vi "Actuator and Pump Control Phases Main Prog.vi"() -> ()   [LabVIEW 2020]
uses:
  Controls/Pump Phases.ctl
  Controls/SImulation Data.ctl
  <vilib>/Instr/_visa.llb/VISA Open Access Mode.ctl
  <vilib>/Instr/_visa.llb/VISA Configure Serial Port (Instr).vi
  <vilib>/Utility/file.llb/Read Delimited Spreadsheet (string).vi
  <vilib>/Utility/file.llb/Write Delimited Spreadsheet (string).vi
  SubVIs/Pump Global Variables.vi
panel:
  in  "Clear Simulation Data":bool
  in  "stop 3":bool
  out "error out 5":errorcluster
  out "VISA resource name out 3":refnum<visa-resource-name>
  out "error out 4":errorcluster
  out "VISA resource name out 2":refnum<visa-resource-name>
  out "Valve error out":errorcluster
  out "Valve resource name out":refnum<visa-resource-name>
  out "read buffer":string
  in  "Volume Dis Update":bool
  out "Dispensed":string
  out "Extracted Numbers":dbl[](array[numeric]) format="%#.6g"
  in  "Simulation data":T1[](array[typedef]) {"Time Stamp" format="%<%.3X>T"}
  out "Elapsed Time (s)":dbl
  out "Time":timestamp=timestamp(3688120494.225 s since 1904-01-01)
  in  "stop 2":bool
  in  "State?":bool
  in  "Pump Phases Path":path
  out "source 2":string
  out "code 2":i32
  out "status 2":bool
  out "source":string
  out "code":i32
  out "status":bool
  in  "Save Simulation Data":bool
  in  "Save Pump Phases":bool
  in  "Load Pump Phases":bool
  in  "Save Basic Param":bool
  out "Complete":bool[](array[boolean])
  out "Busy":bool caption="BUSY"
  in  "Add":bool
  in  "Update":bool
  in  "Delete last":bool
  in  "Delete unselected":bool
  in  "Select":bool[](array[boolean])=[TRUE, TRUE, TRUE, TRUE, TRUE, TRUE, TRUE, TRUE, TRUE, TRUE, TRUE, TRUE, TRUE]
  out "Direction1":string caption="Direction"
  out "Rate1":string caption="Rate"
  out "Target1":string caption="Target"
  in  "RUN":bool
  in  "Serial Reset":bool
  in  "Reset1":bool
  in  "Send":bool
  in  "Units":string(combo)="mm"
  in  "Pump Direction":string(combo)="wdr"
  in  "Incr/Decr Time (S)":dbl
  in  "Diameter (mm)":dbl=20.5 min=0.1 max=50.0
  in  "Array of Pump Phases":T2[](array[typedef]) {"Valve Position" min=0 max=10 step=1; "Pump Rate" format="%#_4g"}
  out "Max rate":dbl format="%#_4g"
  out "Min rate":dbl format="%#_4g"
  in  "Pump Serial Port":refnum<visa-resource-name>="COM1"
  in  "stop":bool
  out "error out 2":cluster{}
  in  "Valve VISA resource name":refnum<visa-resource-name>="COM2"
  out "error out":cluster{}
  in  "Send/read":bool
  in  "Stop":bool=TRUE
  out "Read Buffer":string
  in  "Valve Command":string="/?"
  in  "Valve Control":T3(radio)=enum."SetR1"
  out "Numeric":i32
  out "Bytes at Port":u32
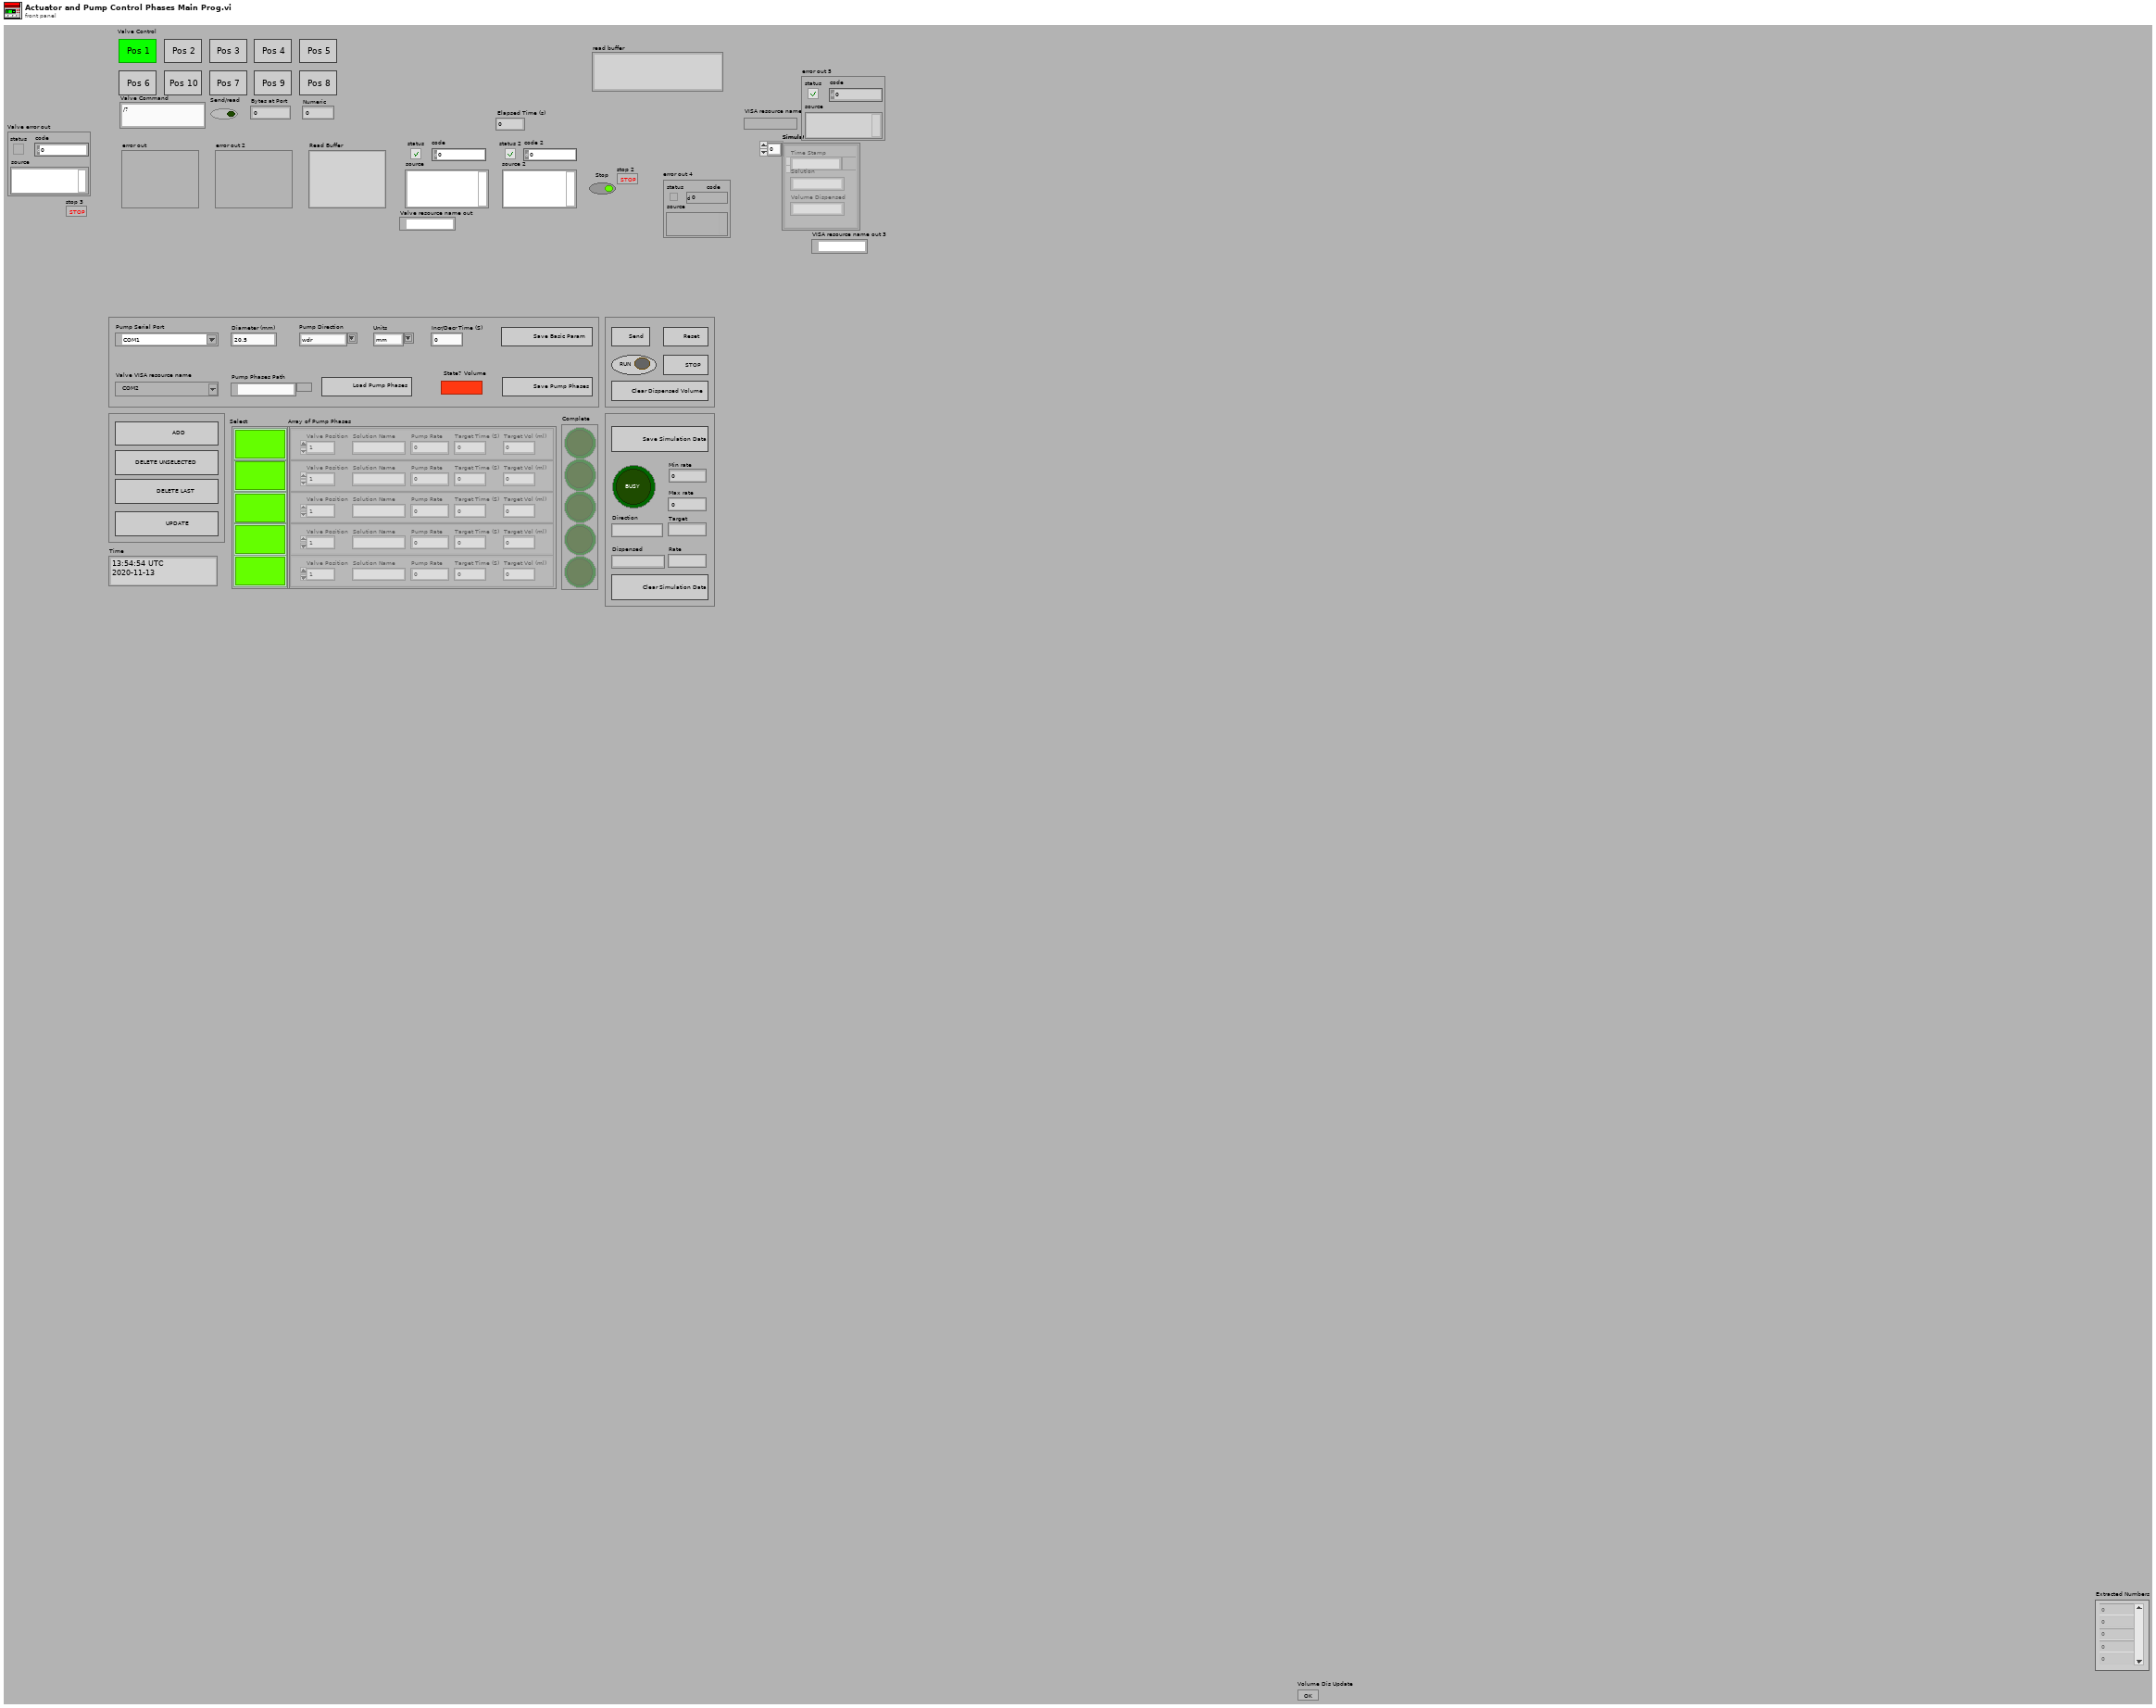
[diagram p1: front panel]
types:
  T1 = typedef "SImulation Data.ctl" = cluster{"Time Stamp":timestamp, "Solution":string, "Volume Dispensed":string}
  T2 = typedef "Pump Phases.ctl" = cluster{"Valve Position":sgl, "Solution Name":string, "Pump Rate":dbl, "Target Time":dbl, "Target Volume":dbl}
  T3 = enum32{"No Selection", "SetR1", "SetR2", "SetR3", "SetR4", "SetR6", "SetR7", "SetR8", "SetR9", "SetR10", "SetR5"}
  T4 = enum8{"Enabled", "Disabled", "Disabled and Grayed Out"}
  T5 = typedef "VISA Open Access Mode.ctl" = u32
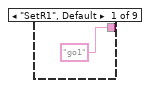
[diagram p2: hidden frame]
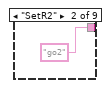
[diagram p3: hidden frame]
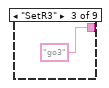
[diagram p4: hidden frame]
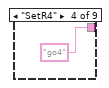
[diagram p5: hidden frame]
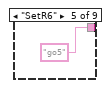
[diagram p6: hidden frame]
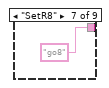
[diagram p7: hidden frame]
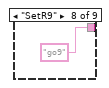
[diagram p8: hidden frame]
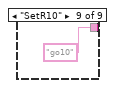
[diagram p9: hidden frame]
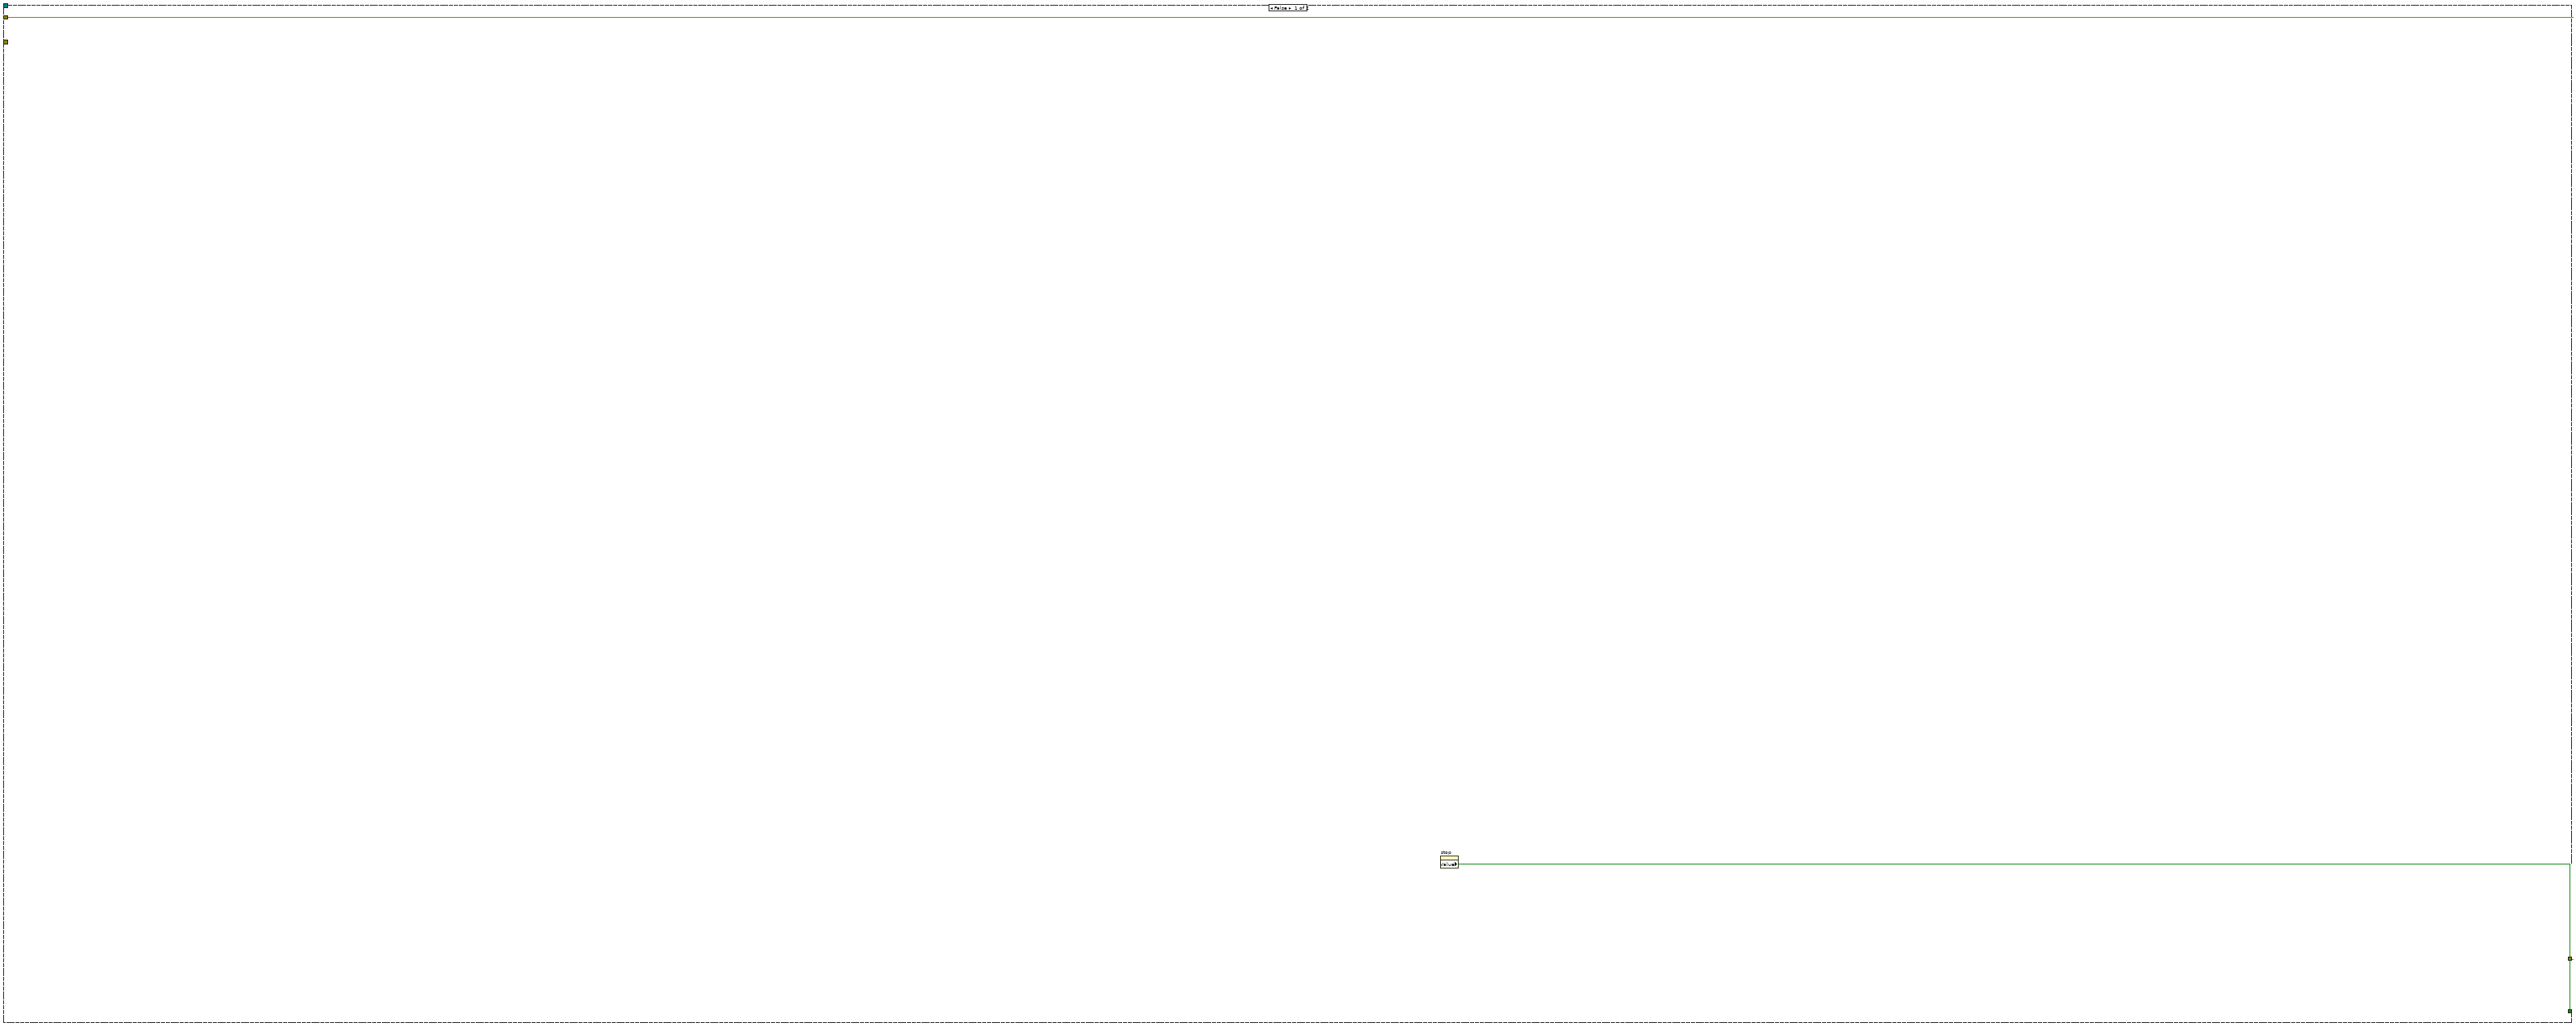
[diagram p13: hidden frame]
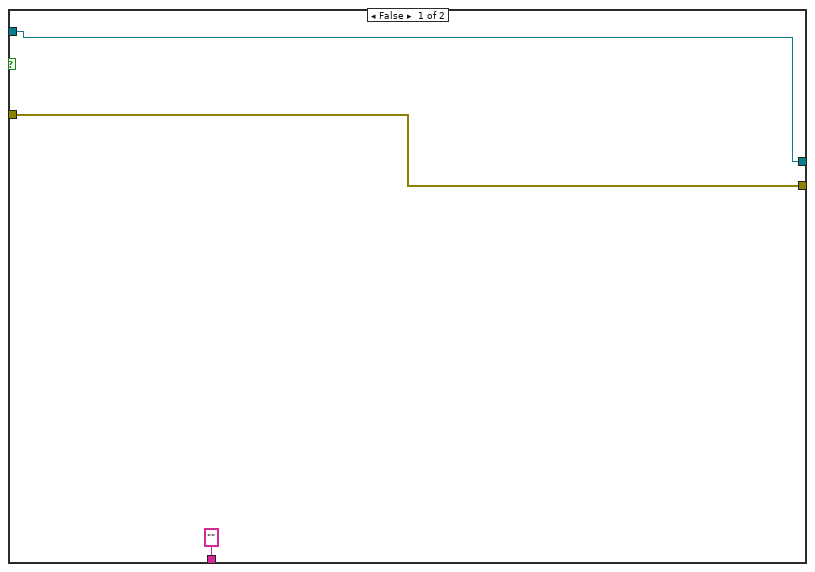
[diagram p14: hidden frame]
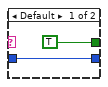
[diagram p15: hidden frame]
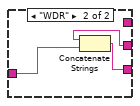
[diagram p16: hidden frame]
diagram:
  n1 = local read "Array of Pump Phases"() -> (w5:T2[])
  n2 = while {
    stop <- "stop 2" stop-if-true
    n3 = call "Elapsed Time"() -> ("Elapsed Time (s)"=→"Elapsed Time (s)":dbl)  [unwired: 12 in, 7 out]
    n4 = Get Date/Time In Seconds() -> (seconds since 1Jan1904=w10:timestamp)
    "Time" <- w10
    n5 = Get Date/Time String(seconds (now)=w10) -> ()  [unwired: 2 in, 2 out]
  }
  n6 = Array Size(array=w5) -> (size(s)=w3:i32)
  n7 = Equal To 0?(x=w3) -> (x = 0?=w4:bool)
  n8 = case shown="True" w4 {
    frame False {
    }
    frame True {
      n9 = Initialize Array(T2 {"Valve Position"=1.0, "Solution Name"="", "Pump Rate"=0.0, "Target Time"=0.0, "Target Volume"=0.0} ("Cluster"), 1 ("dimension size")) -> (w12:T2[])
      n10 = local write "Array of Pump Phases"(w12) -> ()
    }
  }
  n11 = Initialize Array(FALSE, w3) -> (w6:bool[])
  n12 = local write "Complete"(w6) -> ()
  n13 = while {
    tunnel: [w16] -> w8
    tunnel: [w19] -> w2
    tunnel: [w18] -> w1
    stop <- w16 stop-if-true
    w21 = T5 0 items=["VISA Defaults"=0, "Exclusive Lock"=1, "Load Configured Settings"=4] ("Access Mode")
    n14 = VISA Open(access mode=w21, VISA resource name="Valve VISA resource name") -> (VISA resource name=w22:refnum<visa-resource-name>, error out=w24:errorcluster)  [unwired: 3 in]
    n15 = Decimal String To Number(string="9600" ("Baud Rate"), default (0L)=u32 0 ("default (0 I32)")) -> (number=w29:u32)  [unwired: 1 in, 1 out]
    n16 = call-poly "VISA Configure Serial Port"("VISA resource name"="Pump Serial Port", "termination char\n(0xA = '\\n' = LF)"=u8 13 ("termination char\n(0xA = '\\n' = LF)"), "Enable Termination\nChar (T)"=TRUE ("Enable Termination\nChar (T)"), "baud rate (9600)"=w29) -> ("VISA resource name out"=w17:refnum<visa-resource-name>, "error out"=w15:errorcluster)  [unwired: 10 in]
    n17 = call-poly "VISA Configure Serial Port"("VISA resource name"=w22, "Enable Termination\nChar (T)"=FALSE ("Enable Termination\nChar (T)"), "error in (no error)"=w24) -> ("VISA resource name out"=w19:refnum<visa-resource-name>, "error out"=w18:errorcluster)  [unwired: 11 in]
    n18 = Unbundle By Name(w15) -> ("status"=w26:bool)
    n19 = Not(x=w26) -> (.not. x?=w25:bool)
    n20 = case shown="True" w25 {
      tunnel: w17 -> [_ w37]
      tunnel: w15 -> [w35 w42]
      tunnel: [w34 w41] -> w16
      tunnel: [w35 w40] -> w27
      tunnel: w19 -> [_ w39]
      tunnel: w18 -> [_ w38]
      tunnel: w15 -> [_ w36]
      frame False {
        n21 = property on="stop" class="Bool (strict)"() -> ("Value"=w34:bool)  [unwired: 2 in, 2 out]
      }
      frame True {
        n22 = while {
          tunnel: w42 -> [w109]
          tunnel: w37 -> [w110]
          tunnel: [w121] -> w46
          tunnel: [w120] -> w45
          tunnel: ["stop"] -> w41
          tunnel: w39 -> [w111]
          tunnel: w38 -> [w101]
          stop <- w136 stop-if-true
          n23 = Wait Until Next ms Multiple(millisecond multiple=u32 50) -> ()  [unwired: 1 out]
          n24 = global read "Pump Global Variables.vi" "Diameter (mm)"() -> (w126:dbl)
          n25 = case shown="True" "Send" {
            tunnel: w110 -> [w387 w398]
            tunnel: w109 -> [w386 w397]
            tunnel: [w387 w395] -> w108
            tunnel: [w386 w396] -> w107
            tunnel: "Pump Direction" -> [_ w394]
            frame False {
            }
            frame True {
              n26 = flat-sequence {
                tunnel: w398 -> [w403]
                tunnel: w397 -> [w402]
                tunnel: [w400] -> w393
                tunnel: [w399] -> w391
                tunnel: w393 -> [w411]
                tunnel: [w411] -> w392
                tunnel: w391 -> [w410]
                tunnel: [w410] -> w390
                tunnel: w392 -> [w414]
                tunnel: w390 -> [w413]
                tunnel: w394 -> [w412]
                tunnel: [w416] -> w389
                tunnel: [w415] -> w388
                tunnel: [w421] -> w395
                tunnel: [w422] -> w396
                tunnel: w389 -> [w422]
                tunnel: w388 -> [w421]
                frame #0 {
                  n27 = local read "Diameter (mm)"() -> (w405:dbl)
                  n28 = Number To Fractional String(number=w405, precision (6)=i16 2) -> (F-format string=w404:string)  [unwired: 2 in]
                  n29 = Concatenate Strings("dia" ("string"), w404, "\r") -> (w401:string)
                  n30 = VISA Write(VISA resource name=w403, write buffer=w401, error in (no error)=w402) -> (VISA resource name out=w400:refnum<visa-resource-name>, error out=w399:errorcluster)  [unwired: 1 out]
                }
                frame #1 {
                  n31 = Wait (ms)(milliseconds to wait=u32 100) -> ()  [unwired: 1 out]
                }
                frame #2 {
                  n32 = Concatenate Strings("dir" ("string"), w412, "\r") -> (w419:string)
                  n33 = VISA Write(VISA resource name=w414, write buffer=w419, error in (no error)=w413) -> (VISA resource name out=w415:refnum<visa-resource-name>, error out=w416:errorcluster)  [unwired: 1 out]
                }
                frame #3 {
                  n34 = Wait (ms)(milliseconds to wait=u32 100) -> ()  [unwired: 1 out]
                }
              }
            }
          }
          n35 = case shown="True" "Add" {
            frame False {
            }
            frame True {
              n36 = flat-sequence {
                frame #0 {
                  n37 = local read "Array of Pump Phases"() -> (w472:T2[])
                  n38 = Build Array (concatenate)(w472, T2 {"Valve Position"=1.0, "Solution Name"="", "Pump Rate"=0.0, "Target Time"=0.0, "Target Volume"=0.0} ("Cluster")) -> (w470:T2[])
                  n39 = local write "Array of Pump Phases"(w470) -> ()
                }
                frame #1 {
                  n40 = local write "Update"(TRUE) -> ()
                }
              }
            }
          }
          n41 = case shown="True" "Delete last" {
            frame False {
            }
            frame True {
              n42 = flat-sequence {
                frame #0 {
                  n43 = local read "Array of Pump Phases"() -> (w499:T2[])
                  n44 = Delete From Array(array=w499, length=1) -> (array with subset deleted=w500:T2[])  [unwired: 1 in, 1 out]
                  n45 = local write "Array of Pump Phases"(w500) -> ()
                }
                frame #1 {
                  n46 = local write "Update"(TRUE) -> ()
                }
              }
            }
          }
          n47 = case shown="False" "State?" {
            frame False {
              n48 = property on="Target Volume" class="DigNum (strict)"("DisabledEnum"=T4."Enabled" ("Disabled")) -> ()  [unwired: 2 in, 2 out]
              n49 = property on="Target Time" class="DigNum (strict)"("DisabledEnum"=T4."Disabled and Grayed Out" ("Disabled")) -> ()  [unwired: 2 in, 2 out]
            }
            frame True {
              n50 = property on="Target Volume" class="DigNum (strict)"("DisabledEnum"=T4."Disabled and Grayed Out" ("Disabled")) -> ()  [unwired: 2 in, 2 out]
              n51 = property on="Target Time" class="DigNum (strict)"("DisabledEnum"=T4."Enabled" ("Disabled")) -> ()  [unwired: 2 in, 2 out]
            }
          }
          n52 = feedback-in #1("RUN") -> ()
          n53 = feedback #1() -> (w129:bool)  [unwired: 1 in]
          n54 = formula code="r=p*((d/20)**2)*5.1;"("d"=w126, "p"=3.141592653589793) -> ("r"=w134:dbl)
          n55 = global read "Pump Global Variables.vi" "Units 2"() -> (w113:string)
          n56 = case shown="True" "Update" {
            frame False {
            }
            frame True {
              n57 = local read "Array of Pump Phases"() -> (w493:T2[])
              n58 = local write "Update"(FALSE ("Update")) -> ()
              n59 = Array Size(array=w493) -> (size(s)=w492:i32)
              n60 = Greater Than 0?(x=w492) -> (x > 0?=w491:bool)
              n61 = case shown="True" w491 {
                frame False {
                }
                frame True {
                  n62 = local read "Array of Pump Phases"() -> (w498:T2[])
                  n63 = Array Size(array=w498) -> (size(s)=w495:i32)
                  n64 = property on="Select" class="Arr (strict)"("Number of Rows"=w495) -> ()  [unwired: 2 in, 2 out]
                  n65 = property on="Array of Pump Phases" class="Arr (strict)"("Number of Rows"=w495) -> ()  [unwired: 2 in, 2 out]
                  n66 = property on="Complete" class="Arr (strict)"("Number of Rows"=w495) -> ()  [unwired: 2 in, 2 out]
                  n67 = Initialize Array(FALSE, w495) -> (w496:bool[])
                  n68 = local write "Complete"(w496) -> ()
                }
              }
            }
          }
          n69 = case shown="\"mh\"" w113 {
            tunnel: w134 -> [w576 w578 w582 w586 w587]
            tunnel: [w575 w579 w581 w586 w587] -> w131
            frame "mh" {
              n70 = Multiply(x=w576, y=60.0) -> (x*y=w575:dbl)
            }
            frame "um" {
              n71 = Multiply(x=1000.0, y=w578) -> (x*y=w579:dbl)
            }
            frame "uh" {
              n72 = Multiply(x=1000.0, y=60.0) -> (x*y=w585:dbl)
              n73 = Multiply(x=w585, y=w582) -> (x*y=w581:dbl)
            }
            frame Default {
            }
            frame "mm" {
            }
          }
          "Max rate" <- w131
          n74 = disable-structure shown="Disabled" {
            disable-tunnel: w129 -> [w339 _]
            disable-tunnel: "RUN" -> [w336 _]
            frame Disabled {
              n75 = Build Array(w336, w339) -> (w340:bool[])
              n76 = Boolean Array To Number(Boolean array=w340) -> (number=w341:u32)
              n77 = call <vilib>:"Trim Whitespace.vi"("string"="0") -> ("trimmed string"=w338:string)  [unwired: 1 in]
              n78 = case shown="1" w341 {
                tunnel: [w343 w347 w372] -> _
                tunnel: [w342 w346 w371] -> _
                tunnel: _ -> [w343 w351 w370]
                tunnel: _ -> [w342 w350 w369]
                tunnel: w338 -> [_ w345 w366]
                frame 0, Default {
                }
                frame 1 {
                  n79 = local write "Busy"(TRUE) -> ()
                  n80 = Concatenate Strings(w345, "run" ("string"), "\r") -> (w352:string)
                  n81 = flat-sequence {
                    tunnel: w352 -> [w360]
                    tunnel: w351 -> [w359]
                    tunnel: w350 -> [w358]
                    tunnel: [w357] -> w349
                    tunnel: [w356] -> w348
                    tunnel: w349 -> [w364]
                    tunnel: w348 -> [w363]
                    tunnel: [w362] -> w347
                    tunnel: [w361] -> w346
                    frame #0 {
                      n82 = VISA Write(VISA resource name=w359, write buffer=w360, error in (no error)=w358) -> (VISA resource name out=w357:refnum<visa-resource-name>, error out=w356:errorcluster)  [unwired: 1 out]
                      n83 = Wait Until Next ms Multiple(millisecond multiple=u32 200) -> ()  [unwired: 1 out]
                    }
                    frame #1 {
                      n84 = VISA Clear(VISA resource name=w364, error in (no error)=w363) -> (VISA resource name out=w362:refnum<visa-resource-name>, error out=w361:errorcluster)
                    }
                  }
                }
                frame 2 {
                  n85 = local write "Busy"(FALSE ("Busy")) -> ()
                  n86 = Concatenate Strings(w366, "stp" ("string"), "\r") -> (w373:string)
                  n87 = flat-sequence {
                    tunnel: w373 -> [w381]
                    tunnel: w370 -> [w378]
                    tunnel: w369 -> [w377]
                    tunnel: [w380] -> w368
                    tunnel: [w379] -> w367
                    tunnel: [w385] -> w371
                    tunnel: [w382] -> w372
                    tunnel: w368 -> [w384]
                    tunnel: w367 -> [w383]
                    frame #0 {
                      n88 = VISA Write(VISA resource name=w378, write buffer=w381, error in (no error)=w377) -> (VISA resource name out=w380:refnum<visa-resource-name>, error out=w379:errorcluster)  [unwired: 1 out]
                      n89 = Wait Until Next ms Multiple(millisecond multiple=u32 200) -> ()  [unwired: 1 out]
                    }
                    frame #1 {
                      n90 = VISA Clear(VISA resource name=w384, error in (no error)=w383) -> (VISA resource name out=w382:refnum<visa-resource-name>, error out=w385:errorcluster)
                    }
                  }
                }
              }
            }
            frame Enabled {
            }
          }
          n91 = case shown="True" "Clear Simulation Data" {
            frame False {
            }
            frame True {
              n92 = Initialize Array(T1 {"Time Stamp"=timestamp(0 s since 1904-01-01), "Solution"="", "Volume Dispensed"=""} ("Cluster"), 1 ("dimension size")) -> (w140:T1[])
              n93 = local write "Simulation data"(w140) -> ()
            }
          }
          n94 = case shown="True" "Save Simulation Data" {
            frame False {
            }
            frame True {
              n95 = local read "Simulation data"() -> (w144:T1[])
              n96 = for {
                tunnel: [w155] -> w141 mode=indexing
                shift-right: [w154] -> _
                shift-left: 0.0 -> [w153]
                tunnel: w144 -> [w152] mode=indexing
                n97 = Increment(x=w153) -> (x+1=w154:dbl)
                n98 = Number To Decimal String(number=w154) -> (decimal integer string=w156:string)  [unwired: 1 in]
                n99 = Unbundle By Name(w152) -> ("Time Stamp"=w147:timestamp, "Solution"=w150:string, "Volume Dispensed"=w149:string)
                n100 = Concatenate Strings("Phase", w156) -> (w151:string)
                n101 = Format Date/Time String(time format string (%c)="%H:%M:%S", seconds (now)=w147) -> (date/time string=w148:string)  [unwired: 1 in]
                n102 = Build Array(w151, w148, w150, w149) -> (w155:string[])
              }
              n103 = call-poly <vilib>:"Write Delimited Spreadsheet.vi"("format (%s)"="%.13e" ("format (%.3f)"), "2D data"=w141, "transpose? (no:F)"=FALSE) -> ()  [unwired: 11 in, 2 out]
            }
          }
          n104 = case shown="True" "Load Pump Phases" {
            frame False {
            }
            frame True {
              n105 = call-poly <vilib>:"Read Delimited Spreadsheet.vi"("file path (dialog if empty)"="Pump Phases Path", "format (%s)"="%.6e" ("format (%.3f)"), "transpose? (F)"=FALSE ("transpose? (no:F)")) -> ("all rows"=w453:string[][])  [unwired: 7 in, 5 out]
              n106 = for {
                tunnel: [w459] -> w455 mode=indexing
                tunnel: w453 -> [w458] mode=indexing
                n107 = Index Array(array=w458) -> (element #2=w469:string, element #3=w468:string, element #4=w467:string, element #5=w466:string, element #6=w465:string)  [unwired: 6 in, 1 out]
                n108 = Fract/Exp String To Number(string=w469) -> (number=w461:dbl)  [unwired: 3 in, 1 out]
                n109 = Fract/Exp String To Number(string=w467) -> (number=w462:dbl)  [unwired: 3 in, 1 out]
                n110 = Fract/Exp String To Number(string=w466) -> (number=w464:dbl)  [unwired: 3 in, 1 out]
                n111 = Fract/Exp String To Number(string=w465) -> (number=w463:dbl)  [unwired: 3 in, 1 out]
                n112 = Bundle By Name(cluster=T2 {"Valve Position"=1.0, "Solution Name"="", "Pump Rate"=0.0, "Target Time"=0.0, "Target Volume"=0.0} ("Cluster"), "Valve Position"=w461, "Solution Name"=w468, "Pump Rate"=w462, "Target Time"=w464, "Target Volume"=w463) -> (w459:T2)
              }
              n113 = local write "Array of Pump Phases"(w455) -> ()
              n114 = local write "Update"(TRUE) -> ()
            }
          }
          n115 = case shown="True" "Save Pump Phases" {
            frame False {
            }
            frame True {
              n116 = local read "Array of Pump Phases"() -> (w434:T2[])
              n117 = for {
                tunnel: [w448] -> w431 mode=indexing
                shift-right: [w444] -> _
                shift-left: 0.0 -> [w443]
                tunnel: w434 -> [w436] mode=indexing
                n118 = Unbundle By Name(w436) -> ("Valve Position"=w442:sgl, "Solution Name"=w437:string, "Pump Rate"=w441:dbl, "Target Time"=w440:dbl, "Target Volume"=w439:dbl)
                n119 = Increment(x=w443) -> (x+1=w444:dbl)
                n120 = Number To Decimal String(number=w444) -> (decimal integer string=w450:string)  [unwired: 1 in]
                n121 = Concatenate Strings("Phase", w450) -> (w449:string)
                n122 = Number To Fractional String(number=w442) -> (F-format string=w438:string)  [unwired: 3 in]
                n123 = Number To Fractional String(number=w441) -> (F-format string=w447:string)  [unwired: 3 in]
                n124 = Number To Fractional String(number=w440) -> (F-format string=w446:string)  [unwired: 3 in]
                n125 = Number To Fractional String(number=w439) -> (F-format string=w445:string)  [unwired: 3 in]
                n126 = Build Array(w449, w438, w437, w447, w446, w445) -> (w448:string[])
              }
              n127 = call-poly <vilib>:"Write Delimited Spreadsheet.vi"("format (%s)"="%.6e" ("format (%.3f)"), "2D data"=w431, "transpose? (no:F)"=FALSE) -> ()  [unwired: 11 in, 2 out]
            }
          }
          n128 = case shown="True" "Delete unselected" {
            frame False {
            }
            frame True {
              n129 = Two Button Dialog(message="Are you sure you want to delete unselected?") -> (T button?=w474:bool)  [unwired: 2 in]
              n130 = case shown="True" w474 {
                frame False {
                }
                frame True {
                  n131 = local read "Array of Pump Phases"() -> (w477:T2[])
                  n132 = local read "Select"() -> (w481:bool[])
                  n133 = for {
                    tunnel: w477 -> [w485] mode=indexing
                    tunnel: w481 -> [w486] mode=indexing
                    shift-right: [w484] -> w480
                    shift-left: T2[] [] ("Array of Pump Phases") -> [w483]
                    tunnel: [TRUE] -> w479 mode=indexing
                    n134 = case shown="True" w486 {
                      tunnel: w485 -> [_ w490]
                      tunnel: [w487 w489] -> w484
                      tunnel: w483 -> [w487 w488]
                      frame False {
                      }
                      frame True {
                        n135 = Build Array (concatenate)(w488, w490) -> (w489:T2[])
                      }
                    }
                  }
                  n136 = local write "Array of Pump Phases"(w480) -> ()
                  n137 = local write "Select"(w479) -> ()
                  n138 = local write "Update"(TRUE ("Update plot")) -> ()
                }
              }
            }
          }
          n139 = global write "Pump Global Variables.vi" "Pump Direction"("Pump Direction") -> ()
          n140 = case shown="True" "Send" {
            tunnel: [w589 w591] -> w104
            tunnel: w108 -> [w588 w595]
            tunnel: w107 -> [w589 w594]
            tunnel: "Send" -> [_ w592]
            tunnel: [w588 w590] -> w105
            frame False {
            }
            frame True {
              n141 = VISA Clear(VISA resource name=w595, error in (no error)=w594) -> (VISA resource name out=w597:refnum<visa-resource-name>, error out=w596:errorcluster)
              n142 = Build Array("dir", "vol", "rat") -> (w593:string[])
              n143 = case shown="True" w592 {
                tunnel: [w602 w608] -> w590
                tunnel: [w601 w607] -> w591
                tunnel: w593 -> [_ w606]
                tunnel: w597 -> [w602 w605]
                tunnel: w596 -> [w601 w604]
                frame False {
                }
                frame True {
                  n144 = for {
                    N: 3 -> [_]
                    tunnel: w605 -> [w617]
                    tunnel: w604 -> [w616]
                    tunnel: w606 -> [w615] mode=indexing
                    tunnel: [w614] -> w608
                    tunnel: [w613] -> w607
                    i -> [w609]
                    n145 = call "Read Status (SubVI).vi"("error out 2"=w616, "String"=w615, "VISA resource name out 2"=w617) -> ("error out"=w613:errorcluster, "read buffer"=w611:string, "VISA resource name out"=w614:refnum<visa-resource-name>)  [unwired: 1 in]
                    n146 = Search and Replace String(input string=w611, search string="S") -> (result string=w610:string)  [unwired: 6 in, 3 out]
                    n147 = case shown="0" w609 {
                      tunnel: w610 -> [w618 w619 w620 _]
                      frame 0 {
                        "Direction1" <- w618
                      }
                      frame 1 {
                        "Target1" <- w619
                      }
                      frame 2 {
                        "Rate1" <- w620
                      }
                      frame Default {
                      }
                    }
                  }
                }
              }
            }
          }
          n148 = case shown="True" "RUN" {
            tunnel: "Array of Pump Phases" -> [_ w173]
            tunnel: w111 -> [_ w168]
            tunnel: w105 -> [w159 w172]
            tunnel: w104 -> [w158 w171]
            tunnel: [w159 w170] -> w100
            tunnel: [w158 w169] -> w99
            tunnel: w101 -> [_ w163]
            tunnel: "Pump Direction" -> [_ w162]
            tunnel: "stop" -> [_ w160]
            frame False {
            }
            frame True {
              n149 = flat-sequence {
                tunnel: w173 -> [w188]
                tunnel: [w188] -> w167
                tunnel: [w183] -> w164
                tunnel: w163 -> [w183]
                tunnel: ["Diameter (mm)"] -> w161
                tunnel: w172 -> [w201]
                tunnel: w171 -> [w200]
                tunnel: w168 -> [w196]
                tunnel: w167 -> [w203]
                tunnel: [w199] -> w166
                tunnel: [w198] -> w165
                tunnel: w164 -> [w195]
                tunnel: w162 -> [w193]
                tunnel: w161 -> [w192]
                tunnel: w160 -> [w190]
                tunnel: [w334] -> w169
                tunnel: [w335] -> w170
                tunnel: w166 -> [w335]
                tunnel: w165 -> [w334]
                frame #0 {
                  n150 = local read "Time"() -> (w177:timestamp)
                  n151 = local read "Complete"() -> (w187:bool[])
                  n152 = Bundle By Name(cluster=T1 {"Time Stamp"=timestamp(0 s since 1904-01-01), "Solution"="", "Volume Dispensed"=""} ("Cluster"), "Time Stamp"=w177, "Solution"="StartTime", "Volume Dispensed"="00000000000") -> (w180:T1)
                  n153 = Array Size(array=w187) -> (size(s)=w186:i32)
                  n154 = local read "Simulation data"() -> (w179:T1[])
                  n155 = global write "Pump Global Variables.vi" "Diameter (mm)"("Diameter (mm)") -> ()
                  n156 = global write "Pump Global Variables.vi" "Incr/Decr Time (S)"("Incr/Decr Time (S)") -> ()
                  n157 = for {
                    N: w186 -> [_]
                    tunnel: [FALSE] -> w185 mode=indexing
                  }
                  n158 = local write "RUN"(FALSE) -> ()
                  n159 = local write "Complete"(w185) -> ()
                  n160 = Build Array (concatenate)(w179, w180) -> (w174:T1[])
                  n161 = local write "Simulation data"(w174) -> ()
                }
                frame #1 {
                  # "Array of cluster"
                  n162 = global read "Pump Global Variables.vi" "Incr/Decr Time (S)"() -> (w202:dbl)
                  n163 = local read "Simulation data"() -> (w191:T1[])
                  n164 = local read "Complete"() -> (w197:bool[])
                  n165 = global write "Pump Global Variables.vi" "Units 2"("Units") -> ()
                  n166 = for {
                    tunnel: w203 -> [w256] mode=indexing
                    tunnel: [w244] -> w198
                    tunnel: [w251] -> w199
                    tunnel: w193 -> [w253]
                    tunnel: w202 -> [w255]
                    tunnel: "Units" -> [w224]
                    tunnel: w196 -> [w252]
                    tunnel: w201 -> [w225]
                    tunnel: w200 -> [w245]
                    shift-right: [w242] -> _
                    shift-left: w197 -> [w241]
                    tunnel: w195 -> [w226]
                    tunnel: w192 -> [w223]
                    shift-right: [w206] -> _
                    shift-left: w191 -> [w205]
                    tunnel: w190 -> [w204]
                    i -> [w243]
                    n167 = Unbundle By Name(w256) -> ("Valve Position"=w254:sgl, "Solution Name"=w240:string, "Pump Rate"=w230:dbl, "Target Time"=w234:dbl, "Target Volume"=w231:dbl)
                    n168 = flat-sequence {
                      tunnel: w252 -> [w258]
                      tunnel: w253 -> [w263]
                      tunnel: w254 -> [w264]
                      tunnel: [w264] -> w222
                      tunnel: [w263] -> w220
                      tunnel: [w262] -> w218
                      tunnel: w240 -> [w262]
                      tunnel: [w261] -> w216
                      tunnel: w234 -> [w261]
                      tunnel: [w260] -> w214
                      tunnel: w231 -> [w260]
                      tunnel: w230 -> [w259]
                      tunnel: [w259] -> w212
                      tunnel: [w258] -> w210
                      tunnel: [w257] -> w208
                      tunnel: w226 -> [w257]
                      tunnel: w222 -> [w265]
                      tunnel: [w265] -> w221
                      tunnel: w220 -> [w272]
                      tunnel: [w272] -> w219
                      tunnel: w218 -> [w271]
                      tunnel: [w271] -> w217
                      tunnel: w216 -> [w270]
                      tunnel: [w270] -> w215
                      tunnel: w214 -> [w269]
                      tunnel: [w269] -> w213
                      tunnel: w212 -> [w268]
                      tunnel: [w268] -> w211
                      tunnel: w210 -> [w267]
                      tunnel: [w267] -> w209
                      tunnel: w208 -> [w266]
                      tunnel: [w266] -> w207
                      tunnel: w245 -> [w277]
                      tunnel: [w286] -> w248
                      tunnel: w221 -> [w288]
                      tunnel: w219 -> [w282]
                      tunnel: w217 -> [w291]
                      tunnel: [w291] -> w239
                      tunnel: [w290] -> w235
                      tunnel: w215 -> [w290]
                      tunnel: [w289] -> w232
                      tunnel: w213 -> [w289]
                      tunnel: w211 -> [w280]
                      tunnel: [w280] -> w229
                      tunnel: [w279] -> w227
                      tunnel: w209 -> [w285]
                      tunnel: w207 -> [w284]
                      tunnel: w225 -> [w278]
                      tunnel: w224 -> [w276]
                      tunnel: w223 -> [w275]
                      tunnel: w248 -> [w300]
                      tunnel: [w298] -> w247
                      tunnel: [w297] -> w246
                      tunnel: w239 -> [w295]
                      tunnel: [w295] -> w238
                      tunnel: [w294] -> w236
                      tunnel: w235 -> [w294]
                      tunnel: [w293] -> w233
                      tunnel: w232 -> [w293]
                      tunnel: w229 -> [w292]
                      tunnel: [w292] -> w228
                      tunnel: w227 -> [w299]
                      tunnel: w255 -> [w306]
                      tunnel: w224 -> [w315]
                      tunnel: [w314] -> w250
                      tunnel: [w313] -> w249
                      tunnel: w247 -> [w313]
                      tunnel: w246 -> [w314]
                      tunnel: w238 -> [w312]
                      tunnel: [w312] -> w237
                      tunnel: w236 -> [w310]
                      tunnel: w233 -> [w309]
                      tunnel: w228 -> [w308]
                      tunnel: w204 -> [w303]
                      tunnel: [w332] -> w244
                      tunnel: [w331] -> w251
                      tunnel: w250 -> [w330]
                      tunnel: w249 -> [w329]
                      tunnel: w243 -> [w328]
                      tunnel: [w327] -> w242
                      tunnel: w241 -> [w326]
                      tunnel: w237 -> [w325]
                      tunnel: [w320] -> w206
                      tunnel: w205 -> [w319]
                      frame #0 {
                      }
                      frame #1 {
                      }
                      frame #2 {
                        w281 = TRUE
                        n169 = local write "Busy"(w281) -> ()
                        n170 = call "Set Pump Parameters (SubVI).vi"("Units"=w276, "error out 2"=w277, "Target Volume"=0.0, "Flow rate"=w280, "Direction"=w282, "diameter (mm)"=w275, "Send"=w281, "VISA resource name out 2"=w278) -> ()  [unwired: 1 in, 2 out]
                        n171 = call "Set Pump Phases Parameters(SubVI).vi"("Send"=TRUE, "Pump resource in"=w278, "Pump error in"=w277, "Valve Position"=w288, "Pump direction"=w282, "Units"=w276, "Pump rate"=w280, "Valve resource name in"=w285, "Valve error in"=w284) -> ("Pump resource name out"=w286:refnum<visa-resource-name>, "pump error out"=w279:errorcluster, "Valve resource name out"=→"Valve resource name out":refnum<visa-resource-name>, "Valve error out"=→"Valve error out":errorcluster)  [unwired: 3 in]
                      }
                      frame #3 {
                        n172 = Concatenate Strings("run" ("string"), "\r") -> (w296:string)
                        n173 = VISA Write(VISA resource name=w300, write buffer=w296, error in (no error)=w299) -> (VISA resource name out=w298:refnum<visa-resource-name>, error out=w297:errorcluster)  [unwired: 1 out]
                      }
                      frame #4 {
                        n174 = local read "State?"() -> (w307:bool)
                        n175 = call "GetOrCalculate Time from VolumeOrTime.vi"("Units"=w315, "Flow Rate"=w308, "Target Volume"=w309, "Target Time"=w310, "State?"=w307) -> ("Time Output"=w305:dbl)
                        n176 = local write "Volume Dis Update"(TRUE) -> ()
                        n177 = Add(x=w306, y=w305) -> (x+y=w304:dbl)
                        n178 = for {
                          N: w304 -> [_]
                          tunnel: w303 -> [w316]
                          stop <- w316 stop-if-true
                          n179 = Wait (ms)(milliseconds to wait=u32 1000) -> ()  [unwired: 1 out]
                        }
                      }
                      frame #5 {
                        w318 = TRUE
                        n180 = local write "Volume Dis Update"(FALSE) -> ()
                        n181 = local read "Time"() -> (w324:timestamp)
                        n182 = Replace Array Subset(array=w326, new element=w318, index=w328) -> (w327:bool[])
                        n183 = local read "Dispensed"() -> (w323:string)
                        n184 = call "Stop Pumps (SubVI).vi"("error out 2"=w330, "VISA resource name out 2"=w329) -> ("error out"=w332:errorcluster, "VISA resource name out"=w331:refnum<visa-resource-name>)
                        n185 = local write "Complete"(w327) -> ()
                        n186 = call "simulation data VI.vi"("Boolean"=w318, "Volume Dispensed"=w323, "Solution"=w325, "Time Stamp 2"=w324) -> ("Cluster"=w322:T1)
                        n187 = Build Array (concatenate)(w319, w322) -> (w320:T1[])
                        n188 = local write "Simulation data"(w320) -> ()
                      }
                    }
                  }
                }
                frame #2 {
                  n189 = local write "Busy"(FALSE ("Busy")) -> ()
                }
              }
            }
          }
          "VISA resource name out 3" <- w100
          "error out 5" <- w99
          n190 = Multiply(x=w131, y=1.3744e-05) -> (x*y=→"Min rate":dbl)
          n191 = disable-structure shown="Disabled" {
            frame Disabled {
              n192 = case shown="Default" {
                selector: _ -> [_ _ _ _ _]
                frame "mh" {
                  n193 = property on="Pump Rate" class="DigNum (strict)"("Caption.Text"="Pump Rate (ml/h)") -> ()  [unwired: 2 in, 2 out]
                }
                frame "um" {
                  n194 = property on="Pump Rate" class="DigNum (strict)"("Caption.Text"="Pump Rate (ul/m)") -> ()  [unwired: 2 in, 2 out]
                }
                frame "uh" {
                  n195 = property on="Pump Rate" class="DigNum (strict)"("Caption.Text"="Pump Rate (ul/h)") -> ()  [unwired: 2 in, 2 out]
                }
                frame Default {
                }
                frame "mm" {
                  n196 = property on="Pump Rate" class="DigNum (strict)"("Caption.Text"="Pump Rate (ml/m)") -> ()  [unwired: 2 in, 2 out]
                }
              }
            }
            frame Enabled {
            }
          }
          n197 = Build Array("Reset1", FALSE) -> (w125:bool[])
          n198 = Boolean Array To Number(Boolean array=w125) -> (number=w124:u32)
          n199 = case shown="2" w124 {
            selector: w124 -> [w503 w542 _]
            tunnel: w100 -> [w517 w541 w574]
            tunnel: w99 -> [w516 w540 w573]
            tunnel: [w515 w539 w574] -> w121
            tunnel: [w514 w538 w573] -> w120
            frame 1 {
              n200 = Decrement(x=w503) -> (x-1=w504:u32)
              n201 = Number To Decimal String(number=w504) -> (decimal integer string=w505:string)  [unwired: 1 in]
              n202 = Concatenate Strings(w505, "cld" ("string"), "inf" ("string"), "\r") -> (w518:string)
              n203 = Concatenate Strings(w505, "cld" ("string"), "wdr" ("string"), "\r") -> (w506:string)
              n204 = flat-sequence {
                tunnel: w518 -> [w527]
                tunnel: w517 -> [w526]
                tunnel: w516 -> [w525]
                tunnel: [w524] -> w521
                tunnel: [w523] -> w520
                tunnel: w521 -> [w530]
                tunnel: w520 -> [w531]
                tunnel: [w529] -> w511
                tunnel: [w528] -> w510
                tunnel: [w534] -> w514
                tunnel: [w535] -> w515
                tunnel: w511 -> [w536]
                tunnel: w510 -> [w537]
                tunnel: w506 -> [w532]
                frame #0 {
                  n205 = VISA Write(VISA resource name=w526, write buffer=w527, error in (no error)=w525) -> (VISA resource name out=w524:refnum<visa-resource-name>, error out=w523:errorcluster)  [unwired: 1 out]
                  n206 = Wait Until Next ms Multiple(millisecond multiple=u32 200) -> ()  [unwired: 1 out]
                }
                frame #1 {
                  n207 = VISA Clear(VISA resource name=w530, error in (no error)=w531) -> (VISA resource name out=w529:refnum<visa-resource-name>, error out=w528:errorcluster)
                }
                frame #2 {
                  n208 = VISA Write(VISA resource name=w536, write buffer=w532, error in (no error)=w537) -> (VISA resource name out=w535:refnum<visa-resource-name>, error out=w534:errorcluster)  [unwired: 1 out]
                  n209 = Wait Until Next ms Multiple(millisecond multiple=u32 200) -> ()  [unwired: 1 out]
                }
              }
            }
            frame 2 {
              n210 = Decrement(x=w542) -> (x-1=w543:u32)
              n211 = Number To Decimal String(number=w543) -> (decimal integer string=w544:string)  [unwired: 1 in]
              n212 = Concatenate Strings(w544, "cld" ("string"), "inf" ("string"), "\r") -> (w551:string)
              n213 = Concatenate Strings(w544, "cld" ("string"), "wdr" ("string"), "\r") -> (w545:string)
              n214 = flat-sequence {
                tunnel: w551 -> [w562]
                tunnel: w541 -> [w561]
                tunnel: w540 -> [w560]
                tunnel: [w559] -> w556
                tunnel: [w558] -> w555
                tunnel: w556 -> [w565]
                tunnel: w555 -> [w566]
                tunnel: [w564] -> w554
                tunnel: [w563] -> w553
                tunnel: [w569] -> w538
                tunnel: [w570] -> w539
                tunnel: w554 -> [w571]
                tunnel: w553 -> [w572]
                tunnel: w545 -> [w567]
                frame #0 {
                  n215 = VISA Write(VISA resource name=w561, write buffer=w562, error in (no error)=w560) -> (VISA resource name out=w559:refnum<visa-resource-name>, error out=w558:errorcluster)  [unwired: 1 out]
                  n216 = Wait Until Next ms Multiple(millisecond multiple=u32 200) -> ()  [unwired: 1 out]
                }
                frame #1 {
                  n217 = VISA Clear(VISA resource name=w565, error in (no error)=w566) -> (VISA resource name out=w564:refnum<visa-resource-name>, error out=w563:errorcluster)
                }
                frame #2 {
                  n218 = VISA Write(VISA resource name=w571, write buffer=w567, error in (no error)=w572) -> (VISA resource name out=w570:refnum<visa-resource-name>, error out=w569:errorcluster)  [unwired: 1 out]
                  n219 = Wait Until Next ms Multiple(millisecond multiple=u32 200) -> ()  [unwired: 1 out]
                }
              }
            }
            frame Default {
            }
          }
          n220 = Unbundle By Name(w120) -> ("status"=w130:bool)
          n221 = Compound Arithmetic op=OR(w130, "Serial Reset", "stop") -> (w136:bool)
        }
        n222 = while {
          tunnel: w37 -> [w50]
          tunnel: w36 -> [w49]
          stop <- "stop 3" stop-if-true
          n223 = case shown="True" "Volume Dis Update" {
            tunnel: [w53 w74] -> _
            tunnel: [w55 w73] -> _
            tunnel: w49 -> [w55 w72]
            tunnel: ["" ("read buffer") w57] -> w52
            tunnel: w50 -> [w53 w56]
            frame False {
            }
            frame True {
              # "Volume Dispensed"
              n224 = call "Read Status (SubVI).vi"("error out 2"=w72, "String"="dis" ("string"), "VISA resource name out 2"=w56) -> ("error out"=w73:errorcluster, "read buffer"=w57:string, "VISA resource name out"=w74:refnum<visa-resource-name>)  [unwired: 1 in]
              n225 = while {
                shift-left: 0 -> [w80]
                shift-right: [w75] -> _
                tunnel: [w84] -> w58 mode=indexing if=w77
                tunnel: w57 -> [w79]
                stop <- w83 stop-if-true
                w82 = FALSE  # use system decimal point
                w81 = "[-]?[0-9]*[.]?[0-9]*"  # regular expression
                # "Search String for Numbers"
                n226 = Match Pattern(string=w79, regular expression=w81, offset (0)=w80) -> (match substring=w78:string, offset past match=w76:i32)  [unwired: 2 out]
                n227 = Fract/Exp String To Number(use system decimal point (T)=w82, string=w78) -> (number=w84:dbl)  [unwired: 2 in, 1 out]
                n228 = case shown="\"\"" w78 {
                  tunnel: [w86 w88] -> w75
                  tunnel: [TRUE FALSE] -> w77
                  tunnel: w76 -> [w86 w89]
                  frame Default {
                  }
                  frame "" {
                    n229 = Increment(x=w89) -> (x+1=w88:i32)
                  }
                }
                n230 = Less Than 0?(x=w76) -> (x < 0?=w83:bool)
              }
              "Extracted Numbers" <- w58
              n231 = String Length(string=w57) -> (length=w64:i32)
              n232 = property on="Pump Direction" class="CmbBox"() -> ("Value"=w67:string)  [unwired: 2 in, 2 out]
              n233 = Subtract(x=w64, y=2) -> (x-y=w66:i32)
              n234 = String Subset(string=w57, offset (0)=w66, length (rest)=2 ("length (rest)")) -> (substring=w69:string)
              n235 = Index Array(array=w58) -> (element #1=w62:dbl, element #2=w60:dbl)  [unwired: 3 in, 1 out]
              n236 = Number To Fractional String(number=w62) -> (F-format string=w61:string)  [unwired: 3 in]
              n237 = Number To Fractional String(number=w60) -> (F-format string=w59:string)  [unwired: 3 in]
              n238 = case shown="\"INF\", Default" w67 {
                tunnel: [w92 w95] -> w68
                tunnel: w69 -> [w91 w94]
                tunnel: w61 -> [w90 _]
                tunnel: w59 -> [_ w93]
                frame "INF", Default {
                  n239 = Concatenate Strings(w90, w91) -> (w92:string)
                }
                frame "WDR" {
                  n240 = Concatenate Strings(w93, w94) -> (w95:string)
                }
              }
              "Dispensed" <- w68
            }
          }
          "read buffer" <- w52
          n241 = Wait (ms)(milliseconds to wait=u32 100) -> ()  [unwired: 1 out]
        }
        n242 = call "Stop Pumps (SubVI).vi"("error out 2"=w45, "VISA resource name out 2"=w46) -> ("error out"=w43:errorcluster, "VISA resource name out"=w44:refnum<visa-resource-name>)
        n243 = VISA Close(VISA resource name=w44, error in (no error)=w43) -> (error out=w40:errorcluster)
        "VISA resource name out 2" <- w37
        "error out 4" <- w36
      }
    }
    n244 = call <vilib>:"Simple Error Handler.vi"("error in (no error)"=w27) -> ()  [unwired: 4 in, 5 out]
  }
  n245 = disable-structure shown="Disabled" {
    disable-tunnel: w2 -> [w622 _]
    disable-tunnel: w1 -> [w621 _]
    frame Disabled {
      n246 = while {
        tunnel: w622 -> [w627]
        tunnel: w621 -> [w626]
        tunnel: [w628] -> w625
        tunnel: [w629] -> w623
        stop <- "Stop" stop-if-true
        n247 = flat-sequence {
          tunnel: w627 -> [w650]
          tunnel: w626 -> [w649]
          tunnel: [w653] -> w638
          tunnel: [w652] -> w637
          tunnel: "Send/read" -> [w651]
          tunnel: [w682] -> w634
          tunnel: [w683] -> w636
          tunnel: w638 -> [w683]
          tunnel: w637 -> [w682]
          frame #0 {
            n248 = while {
              tunnel: w650 -> [w656]
              tunnel: w649 -> [w655]
              stop <- w654 stop-if-true
              # "Monitor User Interface Events"
              n249 = event shown="[0] \"Valve Control\": Value Change" {
                selector: _ -> [_]
                dyn-events: _ -> [_]
                timeout: _ -> [_]
                tunnel: w656 -> [w659]
                tunnel: w655 -> [w657]
                event "Valve Control": Value Change {
                  n250 = event-data() -> ()  [unwired: 1 in, 1 out]
                  n251 = case shown="\"SetR7\"" "Valve Control" {
                    tunnel: ["go1" "go2" "go3" "go4" "go5" "go7" "go8" "go9" "go10"] -> w661
                    frame "SetR1", Default {
                    }
                    frame "SetR2" {
                    }
                    frame "SetR3" {
                    }
                    frame "SetR4" {
                    }
                    frame "SetR6" {
                    }
                    frame "SetR7" {
                    }
                    frame "SetR8" {
                    }
                    frame "SetR9" {
                    }
                    frame "SetR10" {
                    }
                  }
                  n252 = Concatenate Strings(w661, "\r") -> (w662:string)
                  n253 = VISA Write(VISA resource name=w659, write buffer=w662, error in (no error)=w657) -> ()  [unwired: 3 out]
                }
              }
              n254 = local read "Stop"() -> (w654:bool)
            }
            n255 = case shown="True" w651 {
              tunnel: [w672 w677] -> w653
              tunnel: [w673 w676] -> w652
              tunnel: w650 -> [w673 w675]
              tunnel: w649 -> [w672 w674]
              frame False {
              }
              frame True {
                n256 = Concatenate Strings("Valve Command", "\r") -> (w680:string)
                n257 = VISA Write(VISA resource name=w675, write buffer=w680, error in (no error)=w674) -> (VISA resource name out=w676:refnum<visa-resource-name>, error out=w677:errorcluster)  [unwired: 1 out]
              }
            }
          }
          frame #1 {
            n258 = Wait (ms)(milliseconds to wait=u32 100) -> ()  [unwired: 1 out]
          }
        }
        n259 = while {
          tunnel: w634 -> [w646]
          tunnel: [w645] -> w633
          shift-right: [w647] -> w635
          shift-left: w636 -> [w648]
          shift-right: [w644] -> w632
          shift-left: _ -> [w643]
          i -> [w640]
          stop <- w642 continue-if-true
          n260 = property class="Instr"(reference=w646, error in=w648) -> (reference out=w645:refnum<visa-resource-name>, error out=w647:errorcluster, "Bytes at Port"=w644:u32)
          n261 = Wait (ms)(milliseconds to wait=u32 100) -> ()  [unwired: 1 out]
          n262 = Not Equal?(x=w644, y=w643) -> (x != y?=w642:bool)
          "Numeric" <- w640
        }
        "Bytes at Port" <- w632
        n263 = VISA Read(VISA resource name=w633, byte count=w632, error in (no error)=w635) -> (VISA resource name out=w629:refnum<visa-resource-name>, read buffer=→"Read Buffer":string, error out=w628:errorcluster)  [unwired: 1 out]
      }
      "error out" <- w625
      n264 = VISA Close(VISA resource name=w623) -> (error out=→"error out 2":errorcluster)  [unwired: 1 in]
    }
    frame Enabled {
    }
  }
  n265 = Quit LabVIEW(quit? (T)=w8) -> ()
